vi "LvMPDC_CommandTest.vi"() -> ()   [LabVIEW 2012]
panel:
  out "error out":errorcluster
  in  "btn Enter":bool
  out "Recv Reply":string
  in  "Command":string
  in  "Port":u16=6600
  in  "Server":string
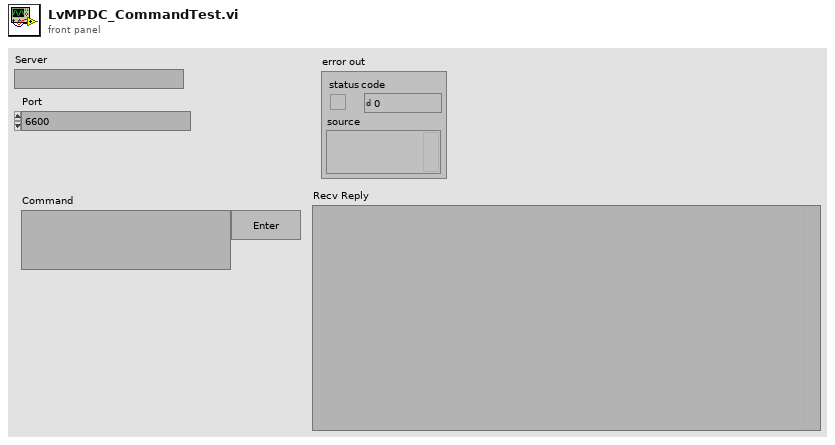
[diagram p1: front panel]
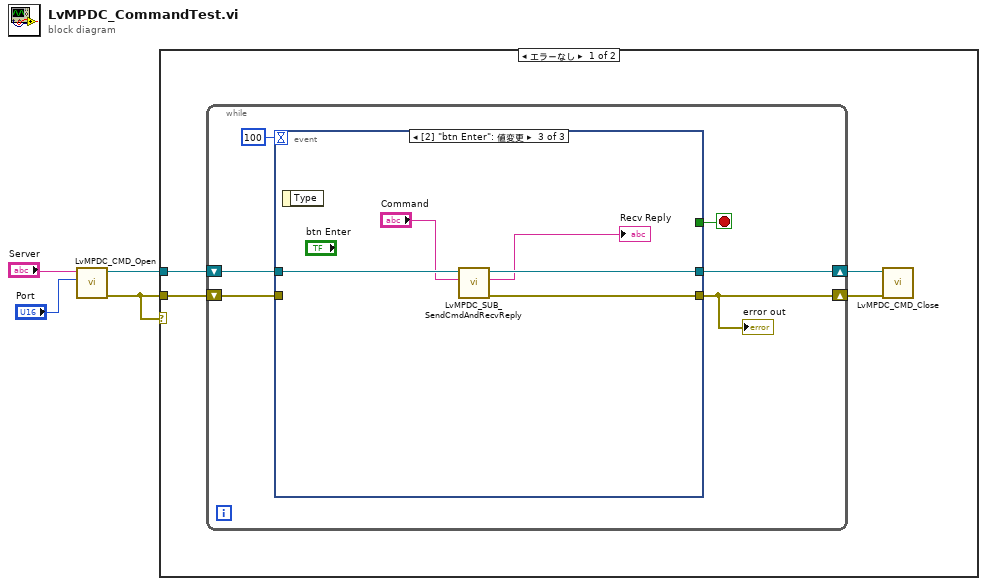
[diagram p0: block diagram]
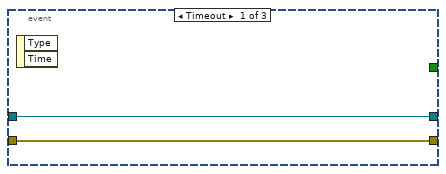
[diagram p2: hidden frame]
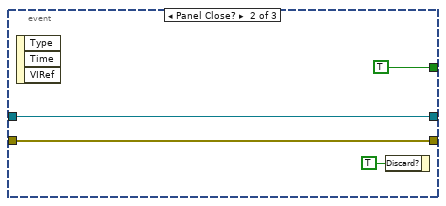
[diagram p3: hidden frame]
diagram:
  n1 = call "LvMPDC_CMD_Open.vi"("Port"="Port", "Server"="Server") -> ("error out"=w3:errorcluster, "Connect ID out"=w4:refnum<k5>)  [unwired: 8 in]
  n2 = case shown="エラーなし" w3 {
    tunnel: w4 -> [w8 _]
    tunnel: w3 -> [w6 _]
    frame No Error {
      n3 = while {
        shift-right: [w12] -> w7
        shift-left: w8 -> [w13]
        shift-right: [w9] -> w5
        shift-left: w6 -> [w11]
        stop <- w10 stop-if-true
        n4 = event shown="[2] \"btn Enter\": 値変更" {
          selector: _ -> [_ _ _]
          dyn-events: _ -> [_ _ _]
          timeout: 100 -> [_ _ _]
          tunnel: w13 -> [w16 w19 w25]
          tunnel: [w16 w19 w24] -> w12
          tunnel: w11 -> [w15 w18 _]
          tunnel: [w15 w18 w23] -> w9
          tunnel: [_ TRUE _] -> w10
          event Timeout {
            n5 = event-data() -> ()  [unwired: 1 in, 2 out]
          }
          event Panel Close? {
            n6 = event-data() -> ()  [unwired: 1 in, 3 out]
            n7 = event-data("Discard?"=TRUE ("破棄?")) -> ()  [unwired: 1 in, 1 out]
          }
          event "btn Enter": Value Change {
            n8 = event-data() -> ()  [unwired: 1 in, 1 out]
            n9 = call "LvMPDC_SUB_SendCmdAndRecvReply.vi"("Command"="Command", "Connect ID"=w25) -> ("error out"=w23:errorcluster, "Reply"=→"Recv Reply":string, "Connect ID out"=w24:refnum<k5>)  [unwired: 7 in]
          }
        }
        "error out" <- w9
      }
      n10 = call "LvMPDC_CMD_Close.vi"("error in (no error)"=w5, "Connect ID"=w7) -> ()  [unwired: 9 in, 1 out]
    }
    frame Error {
    }
  }
